vi "Save Session.vi"(8 "error in (no error)":errorcluster, 11 "Session in":refnum<class "Session.lvclass">) -> (0 "error out":errorcluster, 3 "Session out":refnum<class "Session.lvclass">)   [LabVIEW 2020, in "HTTP Server.lvlib" / "Session.lvclass"]
uses:
  Session.lvclass
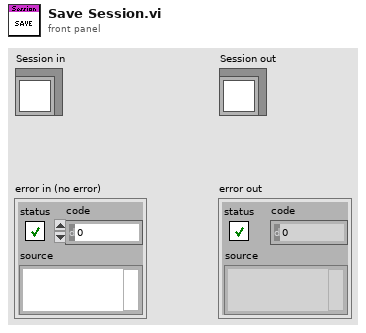
[diagram p1: front panel]
types:
  T1 = enum16{"open", "replace", "create", "open or create", "replace or create", "replace or create with confirmation"}
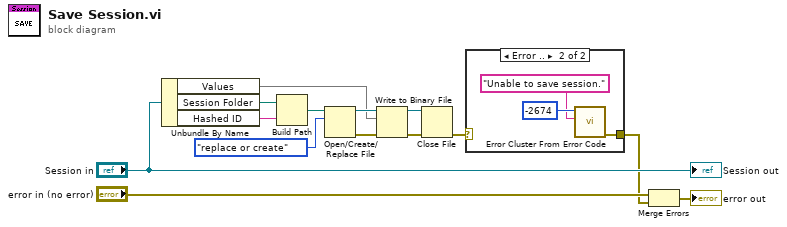
[diagram p0: block diagram]
diagram:
  n1 = Unbundle By Name("Session in") -> ("Values"=w6:map{string, string}, "Session Folder"=w13:path, "Hashed ID"=w11:string)
  n2 = Build Path(base path=w13, name or relative path=w11) -> (appended path=w10:path)
  n3 = Open/Create/Replace File(file path (use dialog)=w10, operation (0:open)=T1."replace or create") -> (refnum out=w8:refnum<file>, error out=w7:errorcluster)  [unwired: 4 in, 1 out]
  n4 = Write to Binary File(file (use dialog)=w8, data=w6, error in=w7) -> (refnum out=w5:refnum<file>, error out=w4:errorcluster)  [unwired: 3 in, 1 out]
  n5 = Close File(refnum=w5, error in=w4) -> (error out=w2:errorcluster)  [unwired: 1 out]
  n6 = case shown="Error .." w2 {
    tunnel: [_ w17] -> w1
    frame No Error {
    }
    frame Error {
      n7 = call <vilib>:"Error Cluster From Error Code.vi"("error message (\"\")"="Unable to save session." ("error message (\"\")"), "error code (0)"=-2674) -> ("error out"=w17:errorcluster)  [unwired: 7 in]
    }
  }
  n8 = Merge Errors("error in (no error)", w1) -> (→"error out":errorcluster)
  "Session out" <- "Session in"
